vi "oa_Extract Waveform Segment (N Channels).vi"(0 "scaled signal [EU]":waveform(dbl)[](array[waveform]), 1 "reset? (True)":bool=TRUE, 5 "pulse positions [s]":dbl[](array[numeric]) format="%.2f", 7 "pulse/revolution (1)":i32=1, 9 "start (rev)":dbl, 11 "error in (no error)":errorcluster) -> (4 "scaled signal [EU]":waveform(dbl)[](array[waveform]), 6 "start":dbl[](array[numeric]), 8 "durations":dbl[](array[numeric]), 10 "duration":dbl, 15 "error out":errorcluster)   [LabVIEW 2017, in "SoundVib_RefDataProcess.lvlib"]
uses:
  <vilib>/addons/Sound and Vibration/Order Analysis/Referece Data Processing/SoundVib_RefDataProcess.lvlib
  <vilib>/Waveform/WDTOps.llb/WDT Get Waveform Subset DBL.vi
  <vilib>/Waveform/WDTOps.llb/WDT Waveform Duration DBL.vi
  <vilib>/Waveform/WDTOps.llb/WDT Append Waveforms DBL.vi
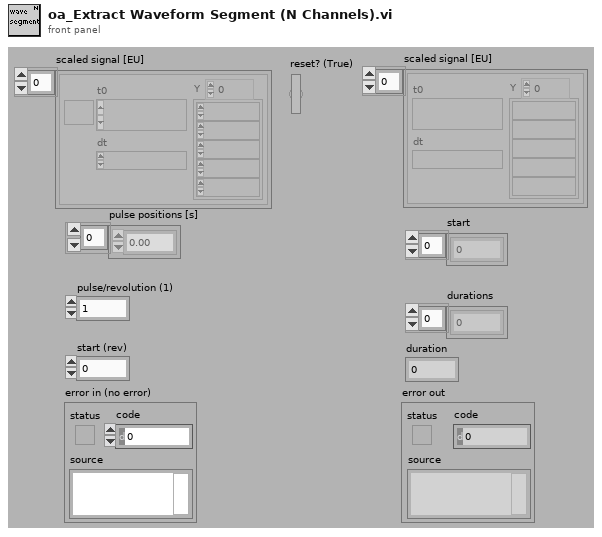
[diagram p1: front panel]
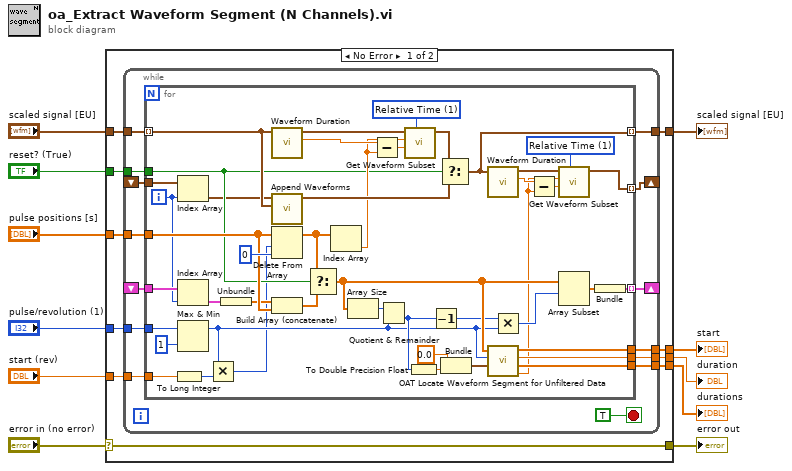
[diagram p0: block diagram]
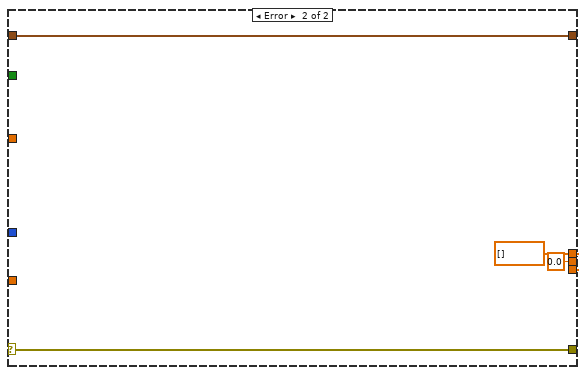
[diagram p2: hidden frame]
diagram:
  n1 = case shown="No Error" "error in (no error)" {
    selector: "error in (no error)" -> [w19 w84]
    tunnel: [w19 w84] -> w10
    tunnel: "scaled signal [EU]" -> [w18 w81]
    tunnel: "reset? (True)" -> [w16 _]
    tunnel: "pulse positions [s]" -> [w20 _]
    tunnel: "pulse/revolution (1)" -> [w21 _]
    tunnel: [w14 w83] -> w5
    tunnel: [w13 0.0 ("duration")] -> w3
    tunnel: [w12 w83] -> w4
    tunnel: [w17 w81] -> w2
    tunnel: "start (rev)" -> [w15 _]
    frame No Error {
      n2 = while {
        tunnel: w21 -> [w35]
        tunnel: w20 -> [w31]
        shift-right: [w33] -> _
        shift-left: _ -> [w32]
        tunnel: w16 -> [w26]
        tunnel: w18 -> [w27]
        shift-right: [w30] -> _
        shift-left: _ -> [w28]
        tunnel: [w29] -> w17
        tunnel: w15 -> [w25]
        tunnel: [w24] -> w14
        tunnel: [w23] -> w13
        tunnel: [w22] -> w12
        stop <- TRUE stop-if-true
        n3 = for {
          tunnel: w35 -> [w79]
          tunnel: [w60] -> w33 mode=indexing
          tunnel: w32 -> [w59]
          tunnel: w31 -> [w75]
          tunnel: [w66] -> w30 mode=indexing
          tunnel: [w65] -> w29 mode=indexing
          tunnel: w28 -> [w62]
          tunnel: w27 -> [w64] mode=indexing
          tunnel: w26 -> [w63]
          tunnel: w25 -> [w38]
          tunnel: [w47] -> w24
          tunnel: [w46] -> w23
          tunnel: [w45] -> w22
          i -> [w56]
          w54 = u16 1 items=["Index", "Relative Time"] ("Mode")
          w72 = u16 1 items=["Index", "Relative Time"] ("Mode")
          n4 = To Long Integer(number=w38) -> (32bit integer=w37:i32)
          n5 = Index Array(array=w62, index=w56) -> (element=w61:waveform(dbl))
          n6 = Index Array(array=w59, index=w56) -> (element=w58:cluster{dbl[]})
          n7 = Max & Min(x=w79, y=1) -> (max(x,y)=w41:i32)  [unwired: 1 out]
          n8 = Multiply(x=w41, y=w37) -> (x*y=w36:i32)
          n9 = Unbundle(w58) -> (w57:dbl[])
          n10 = call-poly <vilib>:"Waveform Duration.vi"("waveform in"=w64) -> ("duration"=w69:dbl, "waveform out"=w73:waveform(dbl))  [unwired: 8 in, 1 out]
          n11 = call-poly <vilib>:"Append Waveforms.vi"("waveform B"=w64, "waveform A"=w61) -> ("waveform out"=w74:waveform(dbl))  [unwired: 8 in, 1 out]
          n12 = Delete From Array(array=w75, length=w36, index=0) -> (array with subset deleted=w70:dbl[])  [unwired: 1 out]
          n13 = Build Array (concatenate)(w57, w75) -> (w77:dbl[])
          n14 = Select(t=w70, s=w63, f=w77) -> (s? t:f=w49:dbl[])
          n15 = Index Array(array=w70) -> (element=w68:dbl)  [unwired: 1 in]
          n16 = Array Size(array=w49) -> (size(s)=w44:i32)
          n17 = Subtract(x=w69, y=w68) -> (x-y=w67:dbl)
          n18 = Quotient & Remainder(x=w44, y=w41) -> (floor(x/y)=w43:i32)  [unwired: 1 out]
          n19 = call-poly <vilib>:"Get Waveform Subset.vi"("start/duration format"=w72, "duration"=w67, "start samples/time"=w68, "waveform in"=w73) -> ("waveform out"=w71:waveform(dbl))  [unwired: 2 in, 3 out]
          n20 = To Double Precision Float(number=w43) -> (double precision float=w42:dbl)
          n21 = Decrement(x=w43) -> (x-1=w40:i32)
          n22 = Select(t=w71, s=w63, f=w74) -> (s? t:f=w65:waveform(dbl))
          n23 = Bundle(0.0, w42) -> (w51:cluster{dbl, dbl})  [unwired: 1 in]
          n24 = call-poly <vilib>:"Waveform Duration.vi"("waveform in"=w65) -> ("duration"=w53:dbl, "waveform out"=w55:waveform(dbl))  [unwired: 8 in, 1 out]
          n25 = call <vilib>:"OAT Locate Waveform Segment for Unfiltered Data.vi"("revolutions to display"=w51, "pulse/revolution (1)"=w41, "pulse positions [s]"=w49) -> ("last point"=w39:dbl, "durations"=w45:dbl[], "duration"=w46:dbl, "start points"=w47:dbl[])  [unwired: 5 in]
          n26 = Multiply(x=w40, y=w41) -> (x*y=w48:i32)
          n27 = Subtract(x=w53, y=w39) -> (x-y=w52:dbl)
          n28 = call-poly <vilib>:"Get Waveform Subset.vi"("start/duration format"=w54, "duration"=w52, "start samples/time"=w39, "waveform in"=w55) -> ("waveform out"=w66:waveform(dbl))  [unwired: 2 in, 3 out]
          n29 = Array Subset(array=w49, index=w48) -> (w78:dbl[])  [unwired: 1 in]
          n30 = Bundle(w78) -> (w60:cluster{dbl[]})  [unwired: 1 in]
        }
      }
    }
    frame Error {
      w83 = dbl[] [] ("start points")
    }
  }
  "error out" <- w10
  "scaled signal [EU]" <- w2
  "start" <- w5
  "durations" <- w4
  "duration" <- w3
